vi "GetBusClass.vi"(8 "ErrorArray In":errorcluster[](array[cluster]), 10 "BusNumber":u8) -> (0 "ErrorArray Out":errorcluster[](array[cluster]), 3 "NISTBus Out":refnum<class "NISTBus.lvclass">)   [LabVIEW 2014, in "Bus.lvlib" / "NISTBus.lvclass"]
uses:
  NISTBus.lvclass
  <vilib>/Utility/error.llb/Error Cluster From Error Code.vi
  <vilib>/ErrorRing/Error Ring.xnode
  <userlib>/NIST/NISTErrorLib/NISTErrorLib.lvlib
  Framework/TestFramework.lvlib
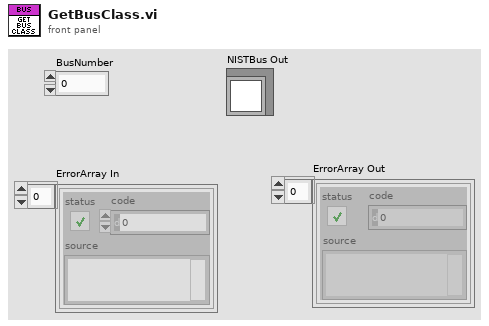
[diagram p1: front panel]
types:
  T1 = typedef "TestFramework.lvlib/clFrameworkData.ctl" = cluster{"NISTBusClassInstances":refnum<class "NISTBus.lvclass">[], "NISTFGenINIFilePaths":path[], "NISTWfrmINIFilePaths":path[]}
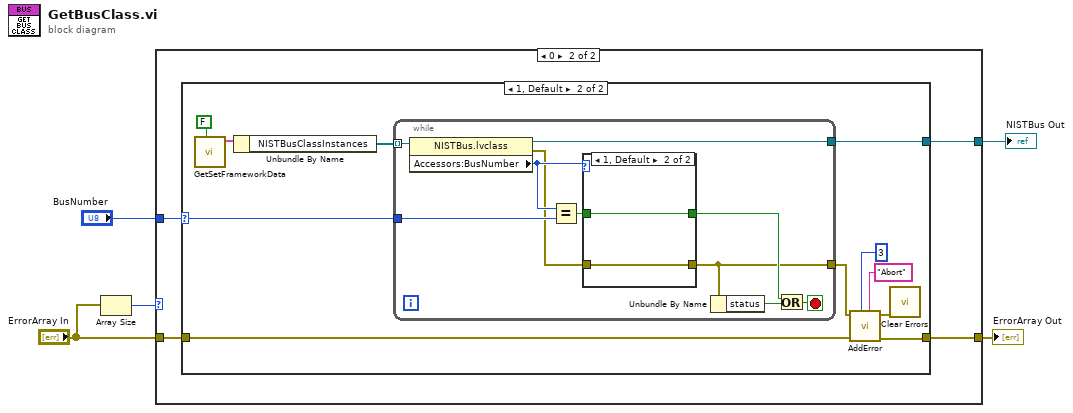
[diagram p0: block diagram]
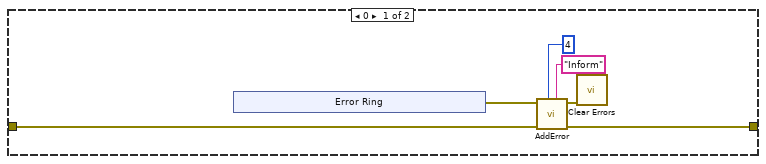
[diagram p3: hidden frame]
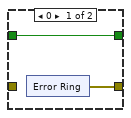
[diagram p4: hidden frame]
diagram:
  n1 = Array Size(array="ErrorArray In") -> (size(s)=w5:i32)
  n2 = case shown="0" w5 {
    tunnel: "ErrorArray In" -> [w6 w10]
    tunnel: [w6 w8] -> w3
    tunnel: "BusNumber" -> [_ w9]
    tunnel: [_ w7] -> w1
    frame 1, Default {
    }
    frame 0 {
      n3 = case shown="1, Default" w9 {
        selector: w9 -> [_ w29]
        tunnel: w10 -> [w11 w23]
        tunnel: [w12 w25] -> w8
        tunnel: [_ w22] -> w7
        frame 0 {
          n4 = xnode "Error Ring"() -> ("error out"=w13:errorcluster)
          n5 = call <userlib>:"AddError.vi"("Severity"="Inform" ("String"), "Priority"=u8 4, "ErrorArray"=w11, "error in (no error)"=w13) -> ("ErrorArray"=w12:errorcluster[], "error out"=w16:errorcluster)  [unwired: 6 in]
          n6 = call <vilib>:"Clear Errors.vi"("error in (no error)"=w16) -> ()  [unwired: 5 in, 2 out]
        }
        frame 1, Default {
          n7 = call "GetSetFrameworkData.vi"("Set (F)"=FALSE) -> ("clFrameworkData Out"=w31:T1)  [unwired: 10 in]
          n8 = Unbundle By Name(w31) -> ("NISTBusClassInstances"=w30:refnum<class "NISTBus.lvclass">[])
          n9 = while {
            tunnel: w30 -> [w42] mode=indexing
            tunnel: w29 -> [w39]
            tunnel: [w35] -> w24
            tunnel: [w33] -> w22
            stop <- w41 stop-if-true
            n10 = property class="NISTBus.lvclass"(reference=w42) -> (reference out=w33:refnum<class "NISTBus.lvclass">, error out=w36:errorcluster, "Accessors:BusNumber"=w40:u8)  [unwired: 1 in]
            n11 = Equal?(x=w40, y=w39) -> (x = y?=w38:bool)
            n12 = case shown="1, Default" w40 {
              tunnel: w38 -> [w44 w50]
              tunnel: [w44 w50] -> w37
              tunnel: w36 -> [_ w51]
              tunnel: [w43 w51] -> w35
              frame 0 {
                n13 = xnode "Error Ring"() -> ("error out"=w43:errorcluster)
              }
              frame 1, Default {
              }
            }
            n14 = Unbundle By Name(w35) -> ("status"=w34:bool)
            n15 = Or(x=w37, y=w34) -> (x .or. y?=w41:bool)
          }
          n16 = call <userlib>:"AddError.vi"("Severity"="Abort" ("String"), "Priority"=u8 3, "ErrorArray"=w23, "error in (no error)"=w24) -> ("ErrorArray"=w25:errorcluster[], "error out"=w28:errorcluster)  [unwired: 6 in]
          n17 = call <vilib>:"Clear Errors.vi"("error in (no error)"=w28) -> ()  [unwired: 5 in, 2 out]
        }
      }
    }
  }
  "NISTBus Out" <- w1
  "ErrorArray Out" <- w3
